vi "1DROISpectrum.vi"(6 "convert output to dB?":bool, 7 "Length of padded array":i32, 9 "Array Subset":T1, 10 "freq (MHz)":dbl format="%.2f", 11 "2-D data array":dbl[][](array[numeric])) -> (1 "df (MHz)":dbl format="%.2f", 3 "power spectrum in dB":dbl[](array[numeric]) format="%.2f")   [LabVIEW 2022 SP3]
uses:
  <vilib>/Analysis/4window.llb/Hamming Window (DBL).vi
  <vilib>/Analysis/2dsp.llb/Real FFT.vi
  <vilib>/Analysis/baseanly.llb/Mean (DBL).vi
  <vilib>/Analysis/4window.llb/AllCosWindow (DBL).vi
  <vilib>/Analysis/NI_AALPro.lvlib
  <vilib>/Analysis/NI_AALBase.lvlib
panel:
  # "Columns represent scan line"
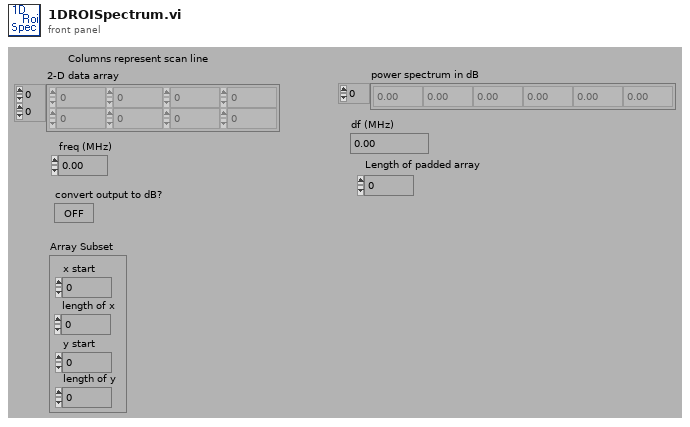
[diagram p1: front panel]
types:
  T1 = cluster{"x start":i32, "length of x":i32, "y start":i32, "length of y":i32}
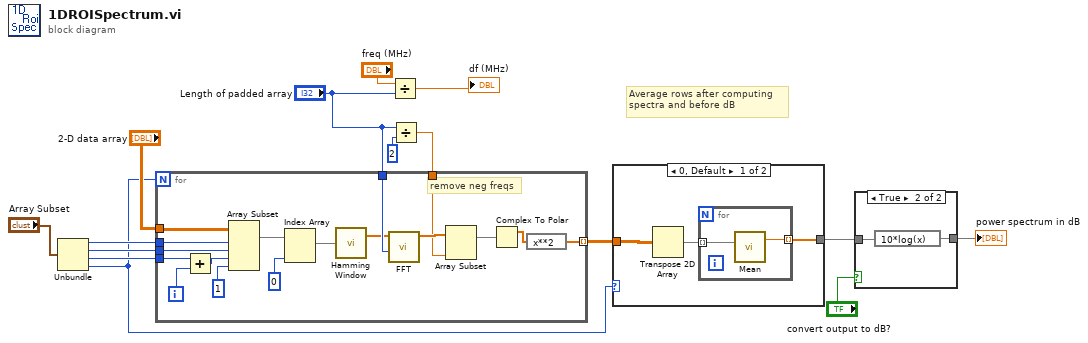
[diagram p0: block diagram]
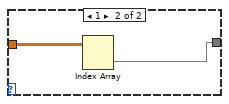
[diagram p2: hidden frame]
diagram:
  # "Average rows after computing\nspectra and before dB"
  n1 = Unbundle("Array Subset") -> ("x start"=w7:i32, "length of x"=w6:i32, "y start"=w8:i32, "length of y"=w5:i32)
  n2 = Divide(x="freq (MHz)", y="Length of padded array") -> (x/y=→"df (MHz)":dbl)
  n3 = Divide(x="Length of padded array", y=2) -> (x/y=w3:dbl)
  n4 = for {
    N: w5 -> [_]
    tunnel: [w20] -> w4 mode=indexing
    tunnel: "2-D data array" -> [w28]
    tunnel: w8 -> [w29]
    tunnel: w7 -> [w27]
    tunnel: w6 -> [w26]
    tunnel: w3 -> [w19]
    tunnel: "Length of padded array" -> [w18]
    i -> [w30]
    # "remove neg freqs"
    n5 = Add(x=w29, y=w30) -> (x+y=w25:i32)
    n6 = Array Subset(array=w28, index (row)=w27, length (row)=w26, index (col)=w25, length (col)=1) -> (w24:dbl[][])
    n7 = Index Array(array=w24, index (col)=0) -> (element=w17:dbl[])  [unwired: 1 in]
    n8 = call-poly <vilib>:"Hamming Window.vi"("X"=w17) -> ("Windowed X"=w16:dbl[])  [unwired: 1 out]
    n9 = call-poly <vilib>:"FFT.vi"("FFT size"=w18, "X"=w16) -> ("FFT {X}"=w32:cdb[])  [unwired: 1 in, 8 out]
    n10 = Array Subset(array=w32, length=w19) -> (w31:cdb[])  [unwired: 1 in]
    n11 = Complex To Polar(r * e^(i*theta)=w31) -> (r=w21:dbl[])  [unwired: 1 out]
    n12 = expression code="x**2"(w21) -> (w20:dbl[])
  }
  n13 = case shown="0, Default" w5 {
    tunnel: [w35 w38] -> w15
    tunnel: w4 -> [w34 w39]
    frame 0, Default {
      n14 = Transpose 2D Array(2D array=w34) -> (transposed array=w33:dbl[][])
      n15 = for {
        tunnel: w33 -> [w36] mode=indexing
        tunnel: [w37] -> w35 mode=indexing
        n16 = call-poly <vilib>:"Mean.vi"("X"=w36) -> ("mean"=w37:dbl)  [unwired: 1 out]
      }
    }
    frame 1 {
      n17 = Index Array(array=w39) -> (element=w38:dbl[])  [unwired: 2 in]
    }
  }
  n18 = case shown="True" "convert output to dB?" {
    tunnel: w15 -> [w40 w42]
    tunnel: [w40 w41] -> w14
    frame False {
    }
    frame True {
      n19 = expression code="10*log(x)"(w42) -> (w41:dbl[])
    }
  }
  "power spectrum in dB" <- w14
